vi "AutobalanceTest.vi"() -> ()   [LabVIEW 2009]
uses:
  Test Utilities/DAQ Read Actions.ctl
panel:
  out "Servo Error vs Command Voltage":cluster{dbl[], dbl[]}[](graph)
  in  "Max Volts":dbl=10.0
  out "Text Output File":path
  out "Result Sample":dbl[](array[numeric])=[9.8]
  in  "milliseconds to wait":u32=10
  in  "Command Voltage Task":refnum<k21>="Command Channels"
  in  "samples per channel":i32=1000
  in  "rate":dbl=100.0 caption="Samples per Second" format="%0.2f"
  in  "Servo Error Task":refnum<k21>="Servo Errors"
  in  "Number of Increments":i32=100
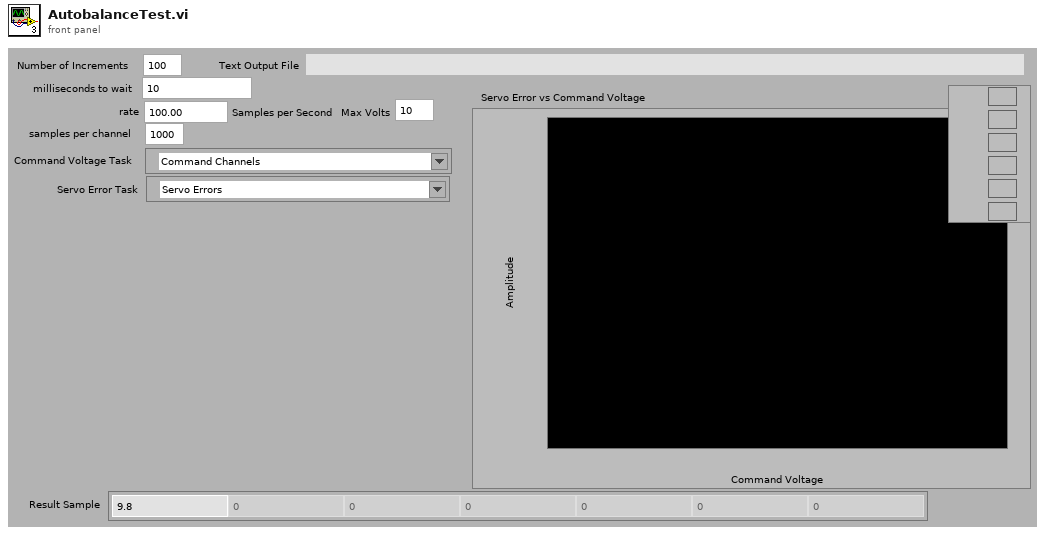
[diagram p1: front panel]
types:
  T1 = typedef "DAQ Read Actions.ctl" = enum16{"Start", "Read", "Stop"}
  T2 = enum16{"open", "replace", "create", "open or create", "replace or create", "replace or create with confirmation"}
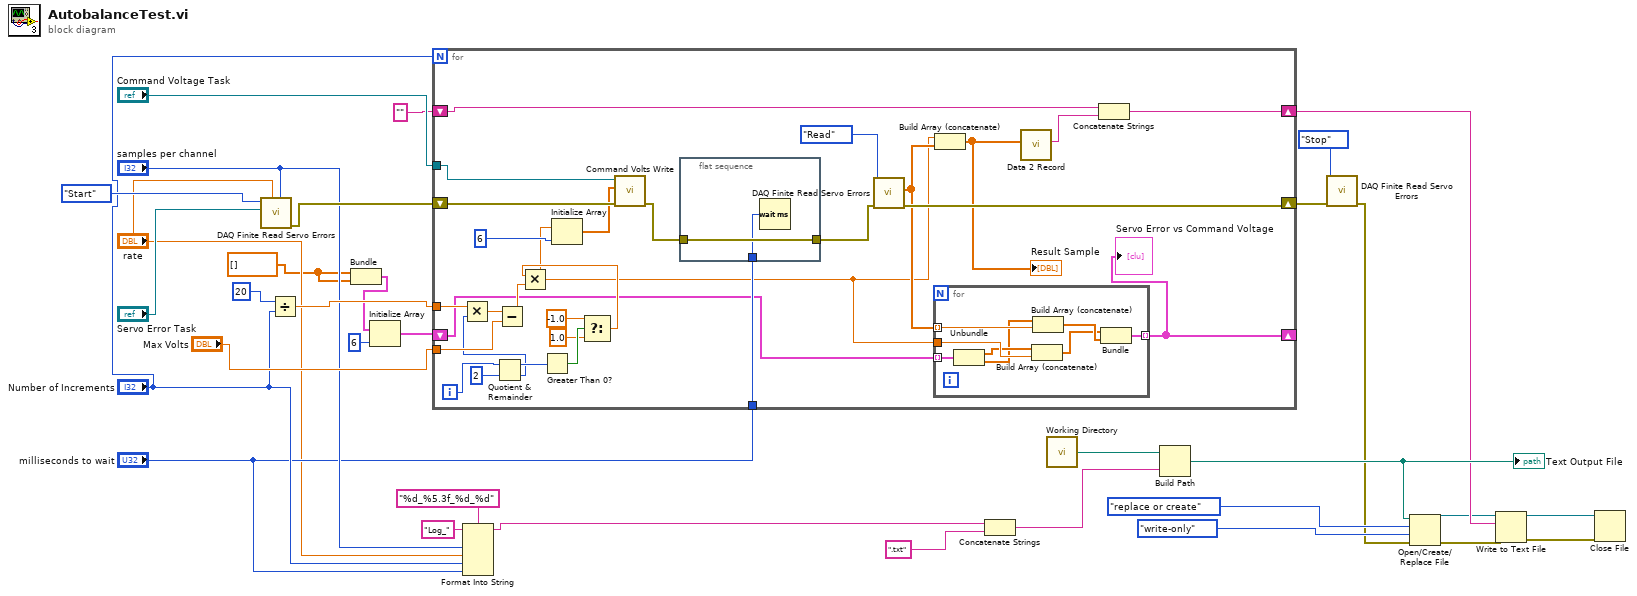
[diagram p0: block diagram]
diagram:
  w3 = dbl[] []
  n1 = call "DAQ Finite Read Servo Errors.vi"("samples per channel"="samples per channel", "rate"="rate", "task/channels in"="Servo Error Task", "Action"=DAQ_Read_Actions."Start") -> ("error out"=w27:errorcluster)  [unwired: 1 in, 6 out]
  n2 = Divide(x=20, y="Number of Increments") -> (x/y=w29:dbl)
  n3 = Bundle(w3, w3) -> (w2:cluster{dbl[], dbl[]})  [unwired: 1 in]
  n4 = Initialize Array(w2, 6 ("dimension size")) -> (w1:cluster{dbl[], dbl[]}[])
  n5 = for {
    N: "Number of Increments" -> [_]
    tunnel: w29 -> [w62]
    tunnel: "Command Voltage Task" -> [w58]
    shift-right: [w55] -> w8
    shift-left: w27 -> [w57]
    tunnel: "milliseconds to wait" -> [w48]
    shift-right: [w49] -> w13
    shift-left: "" -> [w47]
    tunnel: "Max Volts" -> [w60]
    shift-right: [w35] -> _
    shift-left: w1 -> [w34]
    i -> [w46]
    n6 = Quotient & Remainder(x=w46, y=2) -> (x-y*floor(x/y)=w44:i32, floor(x/y)=w39:i32)
    n7 = Multiply(x=w62, y=w39) -> (x*y=w61:dbl)
    n8 = Subtract(x=w61, y=w60) -> (x-y=w38:dbl)
    n9 = Greater Than 0?(x=w44) -> (x > 0?=w43:bool)
    n10 = Select(t=-1.0, s=w43, f=1.0) -> (s? t:f=w40:dbl)
    n11 = Multiply(x=w40, y=w38) -> (x*y=w36:dbl)
    n12 = Initialize Array(w36, 6 ("dimension size")) -> (w52:dbl[])
    n13 = call "Command Volts Write.vi"("error in"=w57, "Command Volts"=w52, "task/channels in"=w58) -> ("error out"=w54:errorcluster)  [unwired: 8 out]
    n14 = flat-sequence {
      tunnel: w54 -> [w72]
      tunnel: [w72] -> w53
      tunnel: w48 -> [w71]
      frame #0 {
        n15 = Wait (ms)(milliseconds to wait=w71) -> ()  [unwired: 1 out]
      }
    }
    n16 = call "DAQ Finite Read Servo Errors.vi"("error in"=w53, "Action"=DAQ_Read_Actions."Read") -> ("error out"=w55:errorcluster, "Average"=w37:dbl[])  [unwired: 3 in, 5 out]
    n17 = for {
      tunnel: w37 -> [w69] mode=indexing
      tunnel: w36 -> [w70]
      tunnel: [w66] -> w35 mode=indexing
      tunnel: w34 -> [w65] mode=indexing
      n18 = Unbundle(w65) -> (w64:dbl[], w63:dbl[])
      n19 = Build Array (concatenate)(w64, w70) -> (w67:dbl[])
      n20 = Build Array (concatenate)(w63, w69) -> (w68:dbl[])
      n21 = Bundle(w67, w68) -> (w66:cluster{dbl[], dbl[]})  [unwired: 1 in]
    }
    "Servo Error vs Command Voltage" <- w35
    n22 = Build Array (concatenate)(w36, w37) -> (w51:dbl[])
    "Result Sample" <- w51
    n23 = call "Data 2 Record.vi"("Data"=w51) -> ("Records"=w50:string)  [unwired: 1 in, 9 out]
    n24 = Concatenate Strings(w47, w50) -> (w49:string)
  }
  n25 = Format Into String(format string="%d_%5.3f_%d_%d", initial string="Log_", "samples per channel", "rate", "Number of Increments", "milliseconds to wait") -> (resulting string=w21:string)  [unwired: 1 in, 1 out]
  n26 = Concatenate Strings(w21, ".txt" ("string")) -> (w16:string)
  n27 = call "Working Directory.vi"() -> ("Path"=w17:path)  [unwired: 1 out]
  n28 = Build Path(base path=w17, name or relative path=w16) -> (appended path=w18:path)
  "Text Output File" <- w18
  n29 = call "DAQ Finite Read Servo Errors.vi"("error in"=w8, "Action"=DAQ_Read_Actions."Stop") -> ("error out"=w7:errorcluster)  [unwired: 3 in, 6 out]
  n30 = Open/Create/Replace File(file path (use dialog)=w18, error in=w7, operation (0:open)=T2."replace or create", access (0:read/write)=enum16{"read/write", "read-only", "write-only"}."write-only") -> (refnum out=w12:refnum<file>, error out=w11:errorcluster)  [unwired: 3 out]
  n31 = Write to Text File(file (use dialog)=w12, text=w13, error in=w11) -> (refnum out=w10:refnum<file>, error out=w9:errorcluster)  [unwired: 2 out]
  n32 = Close File(refnum=w10, error in=w9) -> ()  [unwired: 2 out]
